vi "SHARP_2Y0A02_(SubVI).vi"(10 "Stop":bool, 11 "Calibration Parameters":cluster{"a":dbl, "b":dbl, "c":dbl, "d":dbl}={"a"=4.76809, "b"=2.19854, "c"=3.45456, "d"=0.0655}) -> (0 "error out":errorcluster, 2 "Zeiger":dbl(knob) scale=10.0..150.0)   [LabVIEW 2016]
uses:
  <vilib>/myRIO/Instrument Drivers/Utilities/Utilities.lvlib
  <vilib>/myRIO/Common/Instrument Driver Framework/Utilities/typedefs/Generic FPGA Reference.ctl
  <vilib>/myRIO/Common/Instrument Driver Framework/Utilities/typedefs/myRIO v1.0 Reference.ctl
  <vilib>/myRIO/Common/Instrument Driver Framework/Utilities/typedefs/Hardware Version Enum.ctl
  <vilib>/myRIO/Common/Instrument Driver Framework/Utilities/typedefs/myRIO Generic Hardware Reference.ctl
  <vilib>/myRIO/Express VI/Onboard IO/AI/AI Express VI.xnode
  <vilib>/myRIO/Instrument Drivers/Onboard IO/AI/vis/Read.vi
  <vilib>/myRIO/Instrument Drivers/Onboard IO/AI/AI.lvlib
  <vilib>/myRIO/Common/Instrument Driver Framework/Utilities/typedefs/Analog Scaling Constants.ctl
  <vilib>/myRIO/Common/Instrument Driver Framework/Utilities/typedefs/Analog Scaling Constants List.ctl
  <vilib>/myRIO/Common/Instrument Driver Framework/myRIO v1.0/AI/typedefs/AI Channels Enum.ctl
  <vilib>/myRIO/Common/Instrument Driver Framework/myRIO v1.0/AI/typedefs/AI Channels List.ctl
  <vilib>/myRIO/Instrument Drivers/Onboard IO/AI/typedefs/AI Reference.ctl
  <vilib>/myRIO/Instrument Drivers/Onboard IO/AI/vis/myRIO AI Open.xnode
  <vilib>/myRIO/Common/Instrument Driver Framework/Utilities/vis/Is FPGA Ref Available.vi
  <vilib>/myRIO/Common/Instrument Driver Framework/myRIO v1.0/AI/vis/myRIO v1.1 Open AI.vi
  <vilib>/userdefined/High Color/nirio_resource_hc.ctl
panel:
  out "Numeric":dbl
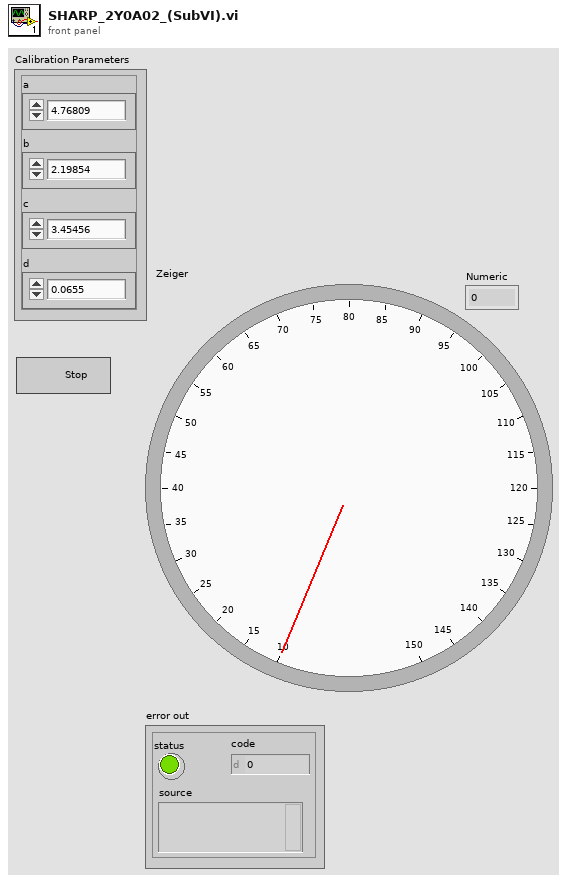
[diagram p1: front panel]
types:
  T1 = typedef "AI.lvlib/AI Reference.ctl" = cluster{"myRIO Reference":T2, "AI Channels List":T6, "AI Scaling Constants List":T8}
  T2 = typedef "myRIO Generic Hardware Reference.ctl" = cluster{"myRIO Model":T3, "myRIO Hardware Reference":T4}
  T3 = typedef "Hardware Version Enum.ctl" = enum16{"Unknown", "myRIO-1900", "myRIO-1950", "roboRIO", "NI ELVIS RIO CM"}
  T4 = typedef "myRIO v1.0 Reference.ctl" = cluster{"Generic FPGA Reference":T5, "Allow multiple opens":bool}
  T5 = typedef "Generic FPGA Reference.ctl" = refnum<k20>
  T6 = typedef "AI Channels List.ctl" = T7[]
  T7 = typedef "AI Channels Enum.ctl" = enum16{"Not Connected", "AudioIn/Left", "AudioIn/Right", "C/AI0", "C/AI1", "A/AI0", "A/AI1", "A/AI2", "A/AI3", "B/AI0", "B/AI1", "B/AI2", "B/AI3", "AI/AI0", "AI/AI1", "AI/AI2", "AI/AI3"}
  T8 = typedef "Analog Scaling Constants List.ctl" = T9[]
  T9 = typedef "Analog Scaling Constants.ctl" = cluster{"LSB Weight (Volts)":dbl, "Offset (Volts)":dbl, "Signed?":bool}
  T10 = typedef "nirio_resource_hc.ctl" = tag
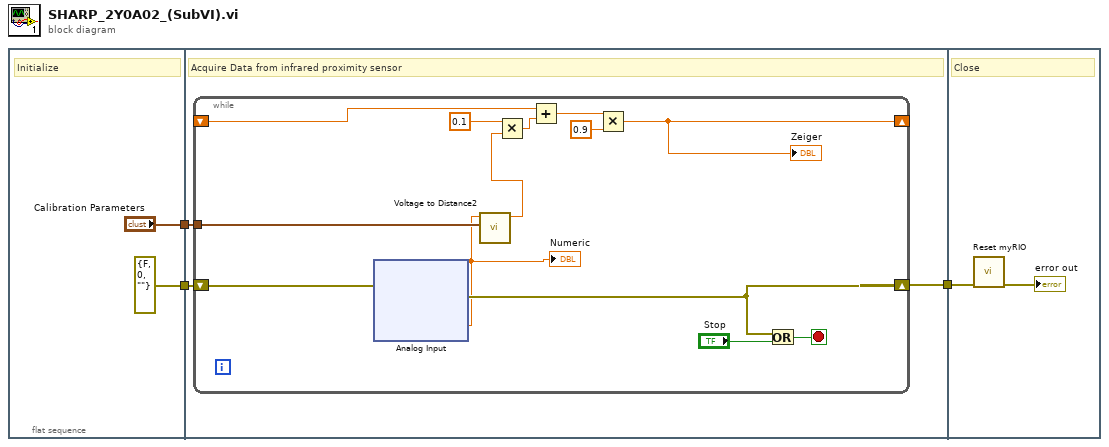
[diagram p0: block diagram]
diagram:
  n1 = flat-sequence {
    tunnel: ["Calibration Parameters"] -> w3
    tunnel: [errorcluster {"status"=FALSE, "code"=0, "source"=""} ("error out")] -> w2
    tunnel: w3 -> [w8]
    tunnel: w2 -> [w7]
    tunnel: [w6] -> w1
    tunnel: w1 -> [w59]
    frame #0 {
      # "Initialize"
    }
    frame #1 {
      # "Acquire Data from infrared proximity sensor"
      n2 = while {
        tunnel: w8 -> [w21]
        shift-right: [w17] -> w6
        shift-left: w7 -> [w18]
        shift-right: [w9] -> _
        shift-left: _ -> [w15]
        stop <- w19 stop-if-true
        n3 = xnode "Analog Input"("error in (no error)"=w18) -> ("B/AI0 (Pin 3)"=w10:dbl, "error out"=w17:errorcluster)
        "Numeric" <- w10
        n4 = call "Voltage to Distance2.vi"("Voltage"=w10, "Calibration Parameters"=w21) -> ("Distance"=w11:dbl)  [unwired: 8 in]
        n5 = Multiply(x=0.1 ("y"), y=w11) -> (x*y=w13:dbl)
        n6 = Add(x=w15, y=w13) -> (x+y=w14:dbl)
        n7 = Multiply(x=w14, y=0.9) -> (x*y=w9:dbl)
        "Zeiger" <- w9
        n8 = Or(x=w17, y="Stop") -> (x .or. y?=w19:bool)
      }
    }
    frame #2 {
      # "Close"
      n9 = call <vilib>:"Reset myRIO.vi"("error in (no error)"=w59) -> ("error out"=→"error out":errorcluster)  [unwired: 10 in]
    }
  }
